vi "unpack12bytes.vi"(7 "Reserved":u16[](array[numeric])=[0, 0, 0, 1] format="%x") -> (4 "number":u32, 6 "number 2":u32, 8 "number 3":u32)   [LabVIEW 2020]
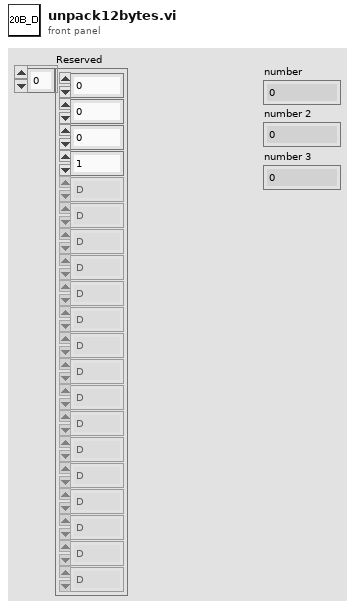
[diagram p1: front panel]
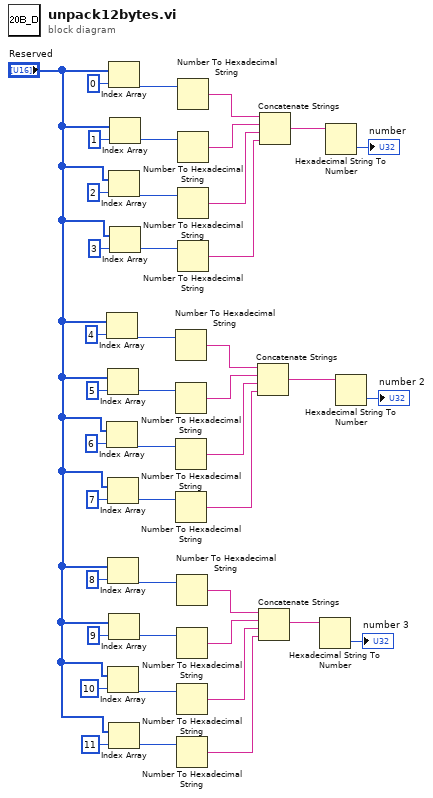
[diagram p0: block diagram]
diagram:
  n1 = Index Array(array="Reserved", index=4) -> (element=w28:u16)
  n2 = Index Array(array="Reserved", index=6) -> (element=w22:u16)
  n3 = Index Array(array="Reserved", index=5) -> (element=w27:u16)
  n4 = Index Array(array="Reserved", index=7) -> (element=w21:u16)
  n5 = Index Array(array="Reserved", index=8) -> (element=w16:u16)
  n6 = Index Array(array="Reserved", index=10) -> (element=w10:u16)
  n7 = Index Array(array="Reserved", index=0) -> (element=w41:u16)
  n8 = Index Array(array="Reserved", index=2) -> (element=w34:u16)
  n9 = Index Array(array="Reserved", index=9) -> (element=w15:u16)
  n10 = Index Array(array="Reserved", index=11) -> (element=w9:u16)
  n11 = Index Array(array="Reserved", index=1) -> (element=w40:u16)
  n12 = Index Array(array="Reserved", index=3) -> (element=w33:u16)
  n13 = Number To Hexadecimal String(2:w28) -> (0:w26:string)  [unwired: 1 in]
  n14 = Number To Hexadecimal String(2:w27) -> (0:w25:string)  [unwired: 1 in]
  n15 = Number To Hexadecimal String(2:w22) -> (0:w20:string)  [unwired: 1 in]
  n16 = Number To Hexadecimal String(2:w21) -> (0:w19:string)  [unwired: 1 in]
  n17 = Number To Hexadecimal String(2:w16) -> (0:w14:string)  [unwired: 1 in]
  n18 = Number To Hexadecimal String(2:w15) -> (0:w13:string)  [unwired: 1 in]
  n19 = Number To Hexadecimal String(2:w10) -> (0:w8:string)  [unwired: 1 in]
  n20 = Number To Hexadecimal String(2:w9) -> (0:w7:string)  [unwired: 1 in]
  n21 = Number To Hexadecimal String(2:w41) -> (0:w39:string)  [unwired: 1 in]
  n22 = Number To Hexadecimal String(2:w40) -> (0:w38:string)  [unwired: 1 in]
  n23 = Number To Hexadecimal String(2:w34) -> (0:w32:string)  [unwired: 1 in]
  n24 = Number To Hexadecimal String(2:w33) -> (0:w31:string)  [unwired: 1 in]
  n25 = Concatenate Strings(w26, w25, w20, w19) -> (w6:string)
  n26 = Concatenate Strings(w14, w13, w8, w7) -> (w5:string)
  n27 = Concatenate Strings(w39, w38, w32, w31) -> (w37:string)
  n28 = Hexadecimal String To Number(string=w5) -> (number=→"number 3":u32)  [unwired: 2 in, 1 out]
  n29 = Hexadecimal String To Number(string=w37) -> (number=→"number":u32)  [unwired: 2 in, 1 out]
  n30 = Hexadecimal String To Number(string=w6) -> (number=→"number 2":u32)  [unwired: 2 in, 1 out]
